vi "checkAck.vi"(8 "error in (no error)":errorcluster, 9 "dataType":T1, 10 "value":variant, 11 "AlCS in":refnum<class "AlCS.lvclass">) -> (0 "error out":errorcluster, 2 "ack":enum16{"CommandAccepted", "CommandRejected"}(ring), 3 "AlCS out":refnum<class "AlCS.lvclass">)   [LabVIEW 2016, in "AlCS.lvclass"]
uses:
  AlCS.lvclass
  Typedefs/data.ctl
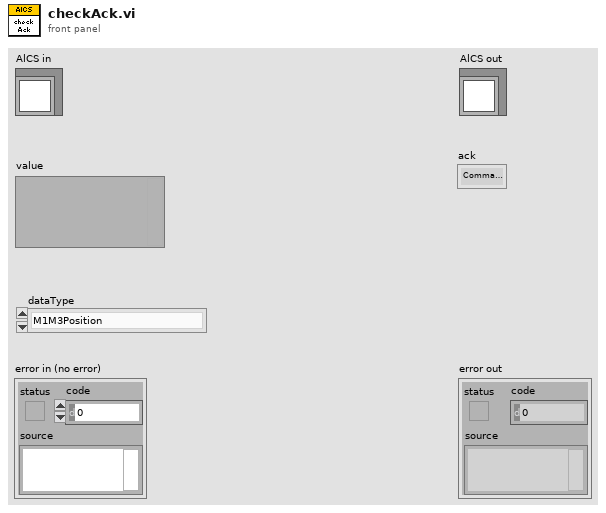
[diagram p1: front panel]
types:
  T1 = typedef "data.ctl" = enum16{"M1M3Position", "M2Position", "CameraPosition", "LaserStatus", "DeviceStatus", "Ack"}
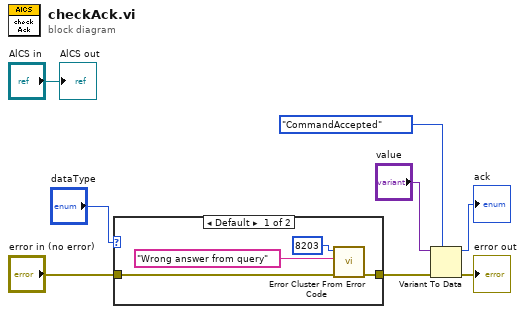
[diagram p0: block diagram]
diagram:
  n1 = case shown="Default" "dataType" {
    tunnel: "error in (no error)" -> [w10 w13]
    tunnel: [w9 w13] -> w5
    frame Default {
      n2 = call <vilib>:"Error Cluster From Error Code.vi"("error in (no error)"=w10, "error message (\"\")"="Wrong answer from query" ("error message (\"\")"), "error code (0)"=8203) -> ("error out"=w9:errorcluster)  [unwired: 6 in]
    }
    frame "Ack" {
    }
  }
  n3 = Variant To Data(error in=w5, type=enum16{"CommandAccepted", "CommandRejected"}."CommandAccepted" ("ack"), Variant="value") -> (data=→"ack":enum16{"CommandAccepted", "CommandRejected"}, error out=→"error out":errorcluster)
  "AlCS out" <- "AlCS in"
